vi "mqttCmdAcknowledge.vi"(0 "_mqtt in":refnum<class "mqttCmdPing.lvclass">, 11 "error in (no error)":errorcluster) -> (4 "_mqtt out":refnum<class "mqttCmdPing.lvclass">, 8 "notification":T1, 15 "error out":errorcluster)   [LabVIEW 2015, in "mqttCmdPing.lvclass"]
uses:
  mqttCmdPing.lvclass
  mqttTypedef/mqttRXdataCluster.ctl
  mqttTypedef/mqttFixedHeaderResponse.ctl
  mqttTypedef/mqttQOSlevel.ctl
  mqttTypedef/mqttMessageType.ctl
  mqttCmd.lvclass/mqttCmd.ctl
  mqttCmd.lvclass
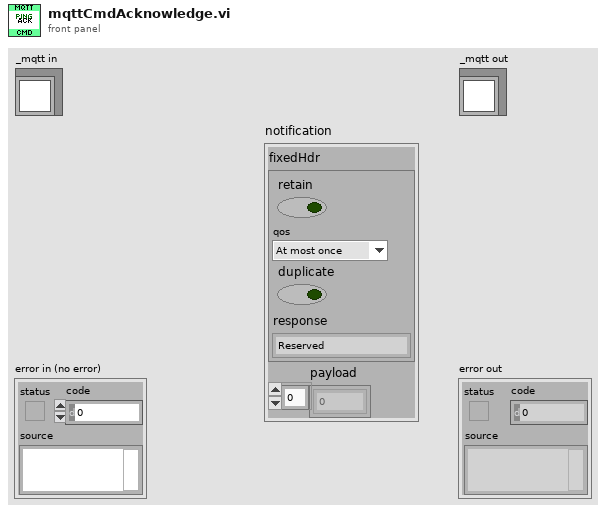
[diagram p1: front panel]
types:
  T1 = typedef "mqttRXdataCluster.ctl" = cluster{"fixedHdr":T2, "payload":u8[]}
  T2 = typedef "mqttFixedHeaderResponse.ctl" = cluster{"retain":bool, "qos":T3, "duplicate":bool, "response":T4}
  T3 = typedef "mqttQOSlevel.ctl" = enum8{"At most once", "At least once", "Exactly once", "Reserved"}
  T4 = typedef "mqttMessageType.ctl" = enum32{"Reserved", "CONNECT", "CONNACK", "PUBLISH", "PUBACK", "PUBREC", "PUBREL", "PUBCOMP", "SUBSCRIBE", "SUBACK", "UNSUBSCRIBE", "UNSUBACK", "PINGREQ", "PINGRESP", "DISCONNECT", "Reserved2"}
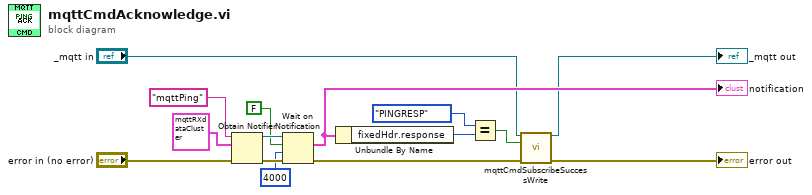
[diagram p0: block diagram]
diagram:
  n1 = Obtain Notifier(name (unnamed)="mqttPing", notification data type=T1 {"fixedHdr"={"retain"=FALSE, "qos"=enum."At most once", "duplicate"=FALSE, "response"=enum."Reserved"}, "payload"=[]} ("notification"), error in (no error)="error in (no error)") -> (notifier out=w12:refnum<notifier>, error out=w15:errorcluster)  [unwired: 1 in, 1 out]
  n2 = Wait on Notification(notifier=w12, ignore previous (F)=FALSE, timeout in ms (-1)=4000, error in (no error)=w15) -> (notification=w8:T1, error out=w4:errorcluster)  [unwired: 2 out]
  "notification" <- w8
  n3 = Unbundle By Name(w8) -> ("fixedHdr.response"=w7:T4)
  n4 = Equal?(x=mqttMessageType."PINGRESP", y=w7) -> (x = y?=w5:bool)
  n5 = call "mqttCmdSubscribeSuccessWrite.vi"("mqttBrokerCommand in"="_mqtt in", "success"=w5, "error in (no error)"=w4) -> ("mqttBrokerCommand out"=→"_mqtt out":refnum<class "mqttCmdPing.lvclass">, "error out"=→"error out":errorcluster)  [unwired: 11 in]
